vi "EEPROM Check ID.vi"(6 "Comparison Mode (F)":bool, 7 "Notes reference":refnum<vi>, 8 "error in (no error)":errorcluster, 9 "Compatible HW version":string, 10 "Top level path":string, 11 "client ptr":u32) -> (0 "error out":errorcluster, 2 "EVM valid? (F)":bool)   [LabVIEW 2010, in "lib1299.lvlib"]
doc: "This VI checks the EEPROM and compares it to the firmware and makes sure the plug-in is operating with compatible hardware.\n\nInputs:\nTop level path - estyx device name of the device top level name\nComparison Mode - FALSE (default): for hardware without EEPROM that is already written\n - TRUE: for hardware with EEPROM already written\nclient ptr - estyx client pointer\nCompatible HW version - version of hardware that this plug-in is compatible with\nerror in - error input cluster\n\nOutputs:\nEVM valid? - FALSE (default): hardware and/or plug-in are not compatible\nerror out - error output cluster"
uses:
  lib1299.lvlib
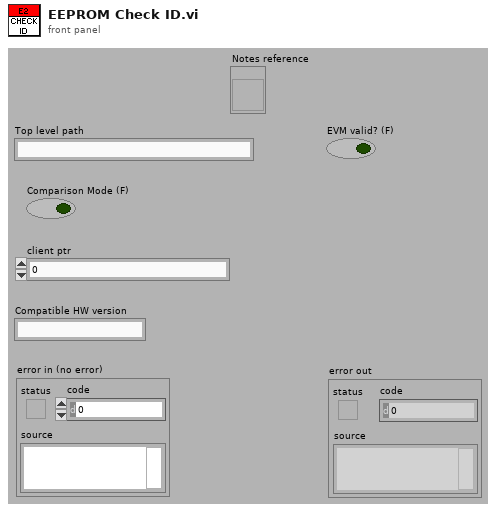
[diagram p1: front panel]
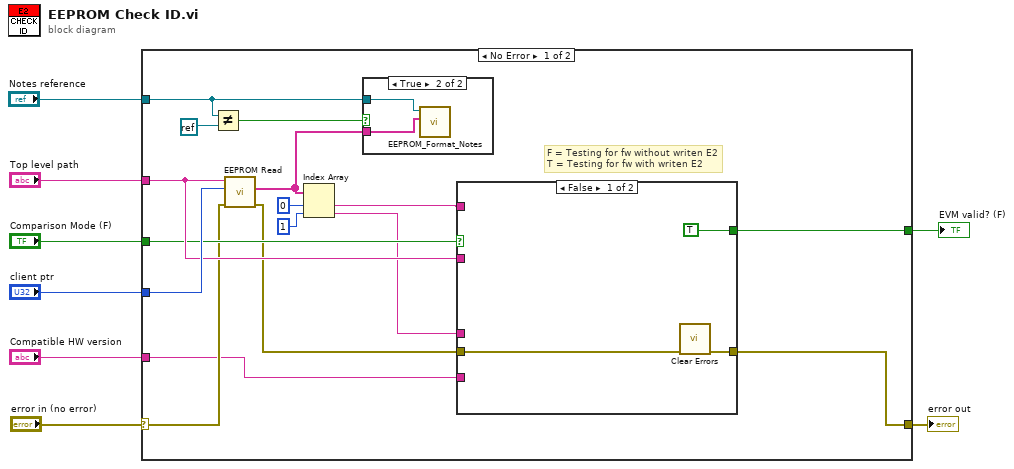
[diagram p0: block diagram]
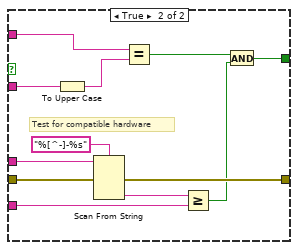
[diagram p3: hidden frame]
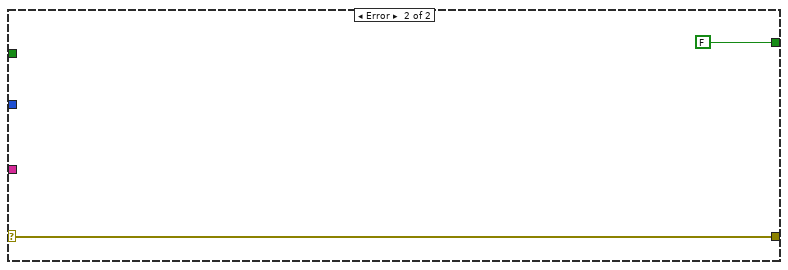
[diagram p4: hidden frame]
diagram:
  n1 = case shown="No Error" "error in (no error)" {
    selector: "error in (no error)" -> [w19 w43]
    tunnel: "client ptr" -> [w24 _]
    tunnel: "Compatible HW version" -> [w15 _]
    tunnel: [w9 FALSE] -> w6
    tunnel: "Top level path" -> [w22 _]
    tunnel: "Comparison Mode (F)" -> [w21 _]
    tunnel: [w16 w43] -> w2
    tunnel: "Notes reference" -> [w12 _]
    frame No Error {
      # "F = Testing for fw without writen E2\nT = Testing for fw with writen E2"
      n2 = Not Equal?(x=w12, y=refnum<k0> refnum) -> (x != y?=w13:bool)
      n3 = call "EEPROM Read .vi"("error in (no error)"=w19, "client ptr"=w24, "Estyx device name"=w22) -> ("error out"=w17:errorcluster, "EEPROM data"=w11:string[])  [unwired: 7 in]
      n4 = Index Array(array=w11, index #1=0 ("index"), index #2=1 ("index")) -> (element #1=w10:string, element #2=w18:string)
      n5 = case shown="True" w13 {
        tunnel: w12 -> [_ w25]
        tunnel: w11 -> [_ w26]
        frame False {
        }
        frame True {
          n6 = call "EEPROM_Format_Notes.vi"("EEPROM data"=w26, "Notes reference"=w25) -> ()  [unwired: 9 in, 1 out]
        }
      }
      n7 = case shown="False" w21 {
        tunnel: w22 -> [_ w41]
        tunnel: w18 -> [_ w39]
        tunnel: w17 -> [w28 w38]
        tunnel: [w27 w37] -> w16
        tunnel: w15 -> [_ w35]
        tunnel: [TRUE w30] -> w9
        tunnel: w10 -> [_ w33]
        frame False {
          n8 = call <vilib>:"Clear Errors.vi"("error in (no error)"=w28) -> ("error out"=w27:errorcluster)  [unwired: 6 in]
        }
        frame True {
          # "Test for compatible hardware"
          n9 = To Upper Case(1:w41) -> (0:w34:string)
          n10 = Scan From String(format string="%[^-]-%s", input string=w39, error in=w38) -> (error out=w37:errorcluster, output 2=w36:string)  [unwired: 4 in, 2 out]
          n11 = Equal?(x=w33, y=w34) -> (x = y?=w32:bool)
          n12 = Greater Or Equal?(x=w36, y=w35) -> (x >= y?=w31:bool)
          n13 = And(x=w32, y=w31) -> (x .and. y?=w30:bool)
        }
      }
    }
    frame Error {
    }
  }
  "EVM valid? (F)" <- w6
  "error out" <- w2
